vi "FP Digital Output.vi"() -> ()   [LabVIEW 2021]
uses:
  Digital Output/Digital Output/Digital Output.lvclass
panel:
  in  "Digital Output.lvlib:Digital Output.lvclass":refnum<class "Digital Output.lvclass">
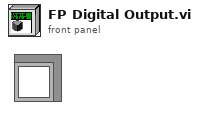
[diagram p1: front panel]
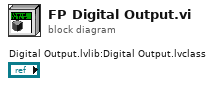
[diagram p0: block diagram]
diagram:
